vi "Create Task.vi"(8 "error in":errorcluster, 10 "Task name":string="PWMOutputTask", 11 "NI PWM Output in":refnum<class "NI PWM Output.lvclass">) -> (0 "error out":errorcluster, 3 "NI PWM Output out":refnum<class "NI PWM Output.lvclass">)   [LabVIEW 2023, in "HardwareAbstractionLayer_LVOOP.lvlib" / "NI PWM Output.lvclass"]
doc: "This VI DAQmx Create Auto Task"
uses:
  NI PWM Output.lvclass
  NI PWM Output.lvclass/NI PWM Output.ctl
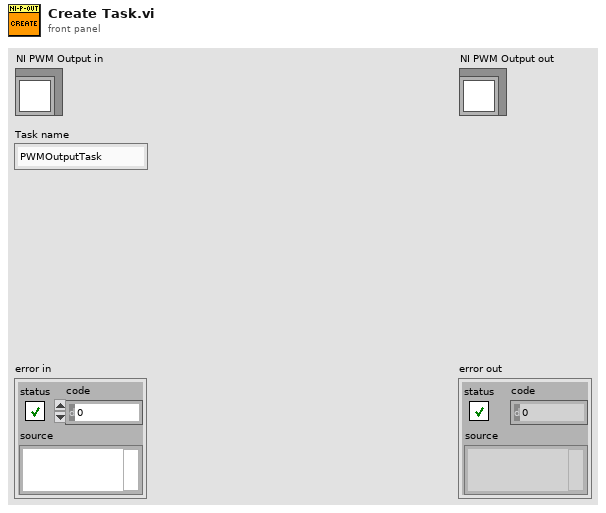
[diagram p1: front panel]
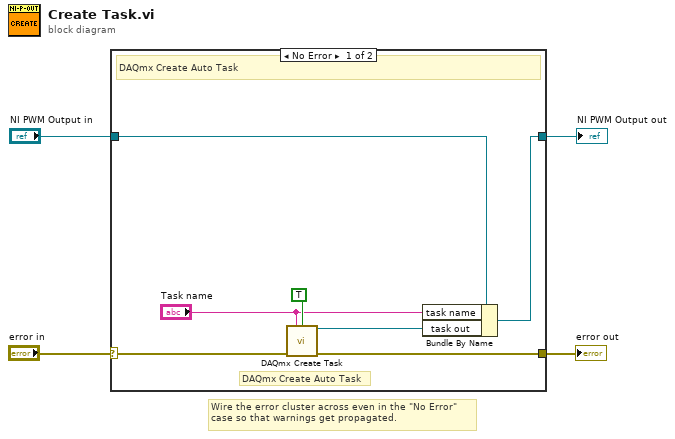
[diagram p0: block diagram]
diagram:
  # "Wire the error cluster across even in the \"No Error\"\ncase so that warnings get propagated."
  n1 = case shown="No Error" "error in" {
    selector: "error in" -> [w11 w13]
    tunnel: [w10 w13] -> w3
    tunnel: [w8 w12] -> w1
    tunnel: "NI PWM Output in" -> [w9 w12]
    frame No Error {
      # "DAQmx Create Auto Task"
      # "DAQmx Create Auto Task"
      n2 = call <vilib>:"DAQmx Create Task.vi"("new task name"="Task name", "auto cleanup"=TRUE, "error in"=w11) -> ("task out"=w7:refnum<k21>, "error out"=w10:errorcluster)  [unwired: 11 in]
      n3 = Bundle By Name(cluster=w9, "task name"="Task name", "task out"=w7) -> (w8:refnum<class "NI PWM Output.lvclass">)
    }
    frame Error {
    }
  }
  "error out" <- w3
  "NI PWM Output out" <- w1
